vi "AuMT8852B Script Name.vi"(5 "Name (\"\")":string, 7 "Set/Get (Set)":enum16{"Set", "Get"}(ring), 8 "error in (no error)":errorcluster, 10 "Script (3)":i32=1, 11 "VISA session":refnum<visa-resource-name>) -> (0 "error out":errorcluster, 2 "error code":i32, 3 "VISA session out":refnum<visa-resource-name>, 4 "Name out":string)   [LabVIEW 2017]
doc: "Anritsu MT8852B Bluetooth Tester\n\nSets the script's display name.\n\nINPUTS\nSet/Get - whether the value is being sent to or retrieved from the instrument.\nScript - which script's name is being written or read. Scripts 1 and 2 are read-only; 3-10 are read-write.\nName - name (16 characters or less) to assign to the script.\n\nOUTPUTS\nName out - the script's current name."
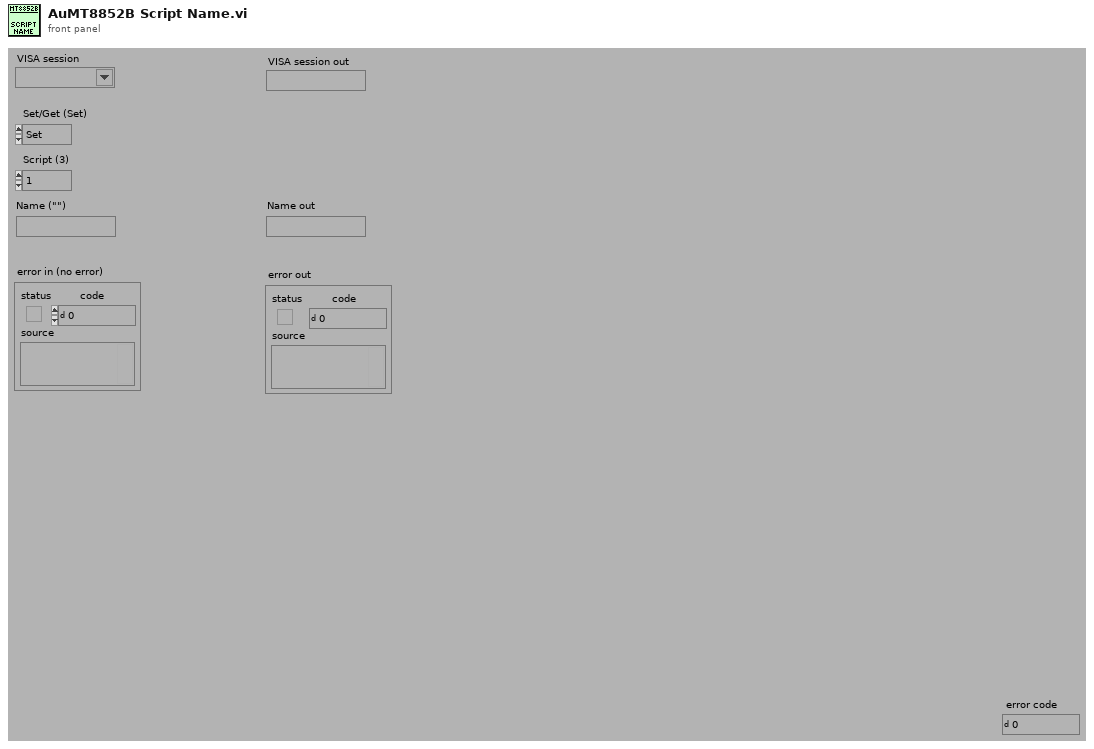
[diagram p1: front panel]
types:
  T1 = enum16{"Simulate", "Range check", "Cache", "Query instrument status"}
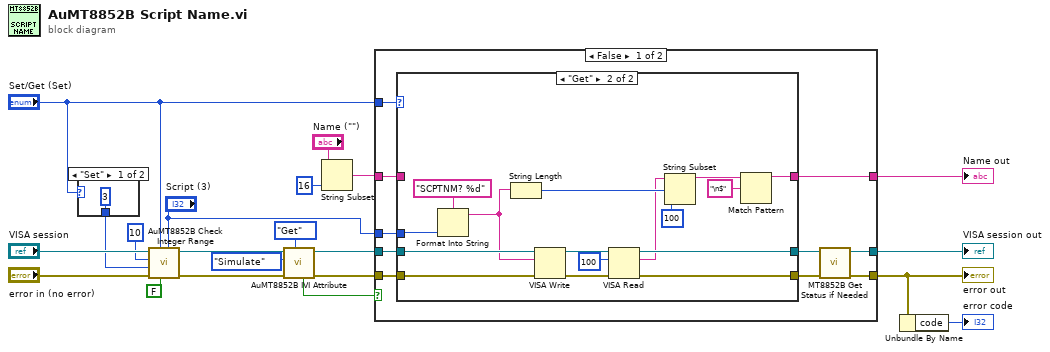
[diagram p0: block diagram]
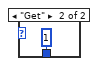
[diagram p2: hidden frame]
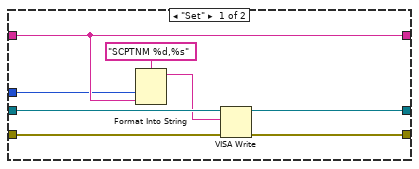
[diagram p3: hidden frame]
diagram:
  n1 = case shown="\"Set\"" "Set/Get (Set)" {
    tunnel: [3 1] -> w16
    frame "Set" {
    }
    frame "Get" {
    }
  }
  n2 = call <instrlib>:"AuMT8852B Check Integer Range.vi"("Value (0)"="Script (3)", "Check IVI flag first? (T)"=FALSE, "Set/Get (Set)"="Set/Get (Set)", "error in (no error)"="error in (no error)", "Lower limit (-1)"=w16, "Upper limit (1)"=10, "VISA session"="VISA session") -> ("error out"=w12:errorcluster, "VISA session out"=w15:refnum<visa-resource-name>)  [unwired: 3 in]
  n3 = call <instrlib>:"AuMT8852B IVI Attribute.vi"("Set/Get (Set)"=enum16{"Set", "Get"}."Get", "error in (no error)"=w12, "Flag (Simulate)"=T1."Simulate", "VISA session"=w15) -> ("error out"=w13:errorcluster, "VISA session out"=w14:refnum<visa-resource-name>, "Value out"=w9:bool)  [unwired: 5 in]
  n4 = String Subset(string="Name (\"\")", length (rest)=16 ("length (rest)")) -> (substring=w6:string)  [unwired: 1 in]
  n5 = case shown="False" w9 {
    tunnel: "Set/Get (Set)" -> [w33 _]
    tunnel: w6 -> [w32 w60]
    tunnel: [w25 w58] -> w2
    tunnel: [w26 w59] -> w21
    tunnel: w14 -> [w31 w59]
    tunnel: w13 -> [w30 w58]
    tunnel: [w29 w60] -> w20
    tunnel: "Script (3)" -> [w24 _]
    frame False {
      n6 = case shown="\"Get\"" w33 {
        tunnel: [w38 w51] -> w27
        tunnel: w32 -> [w35 _]
        tunnel: [w39 w52] -> w28
        tunnel: w31 -> [w41 w57]
        tunnel: w30 -> [w40 w56]
        tunnel: [w35 w43] -> w29
        tunnel: w24 -> [w34 w49]
        frame "Set" {
          n7 = Format Into String(format string="SCPTNM %d,%s" ("Format String"), w34, w35) -> (resulting string=w36:string)  [unwired: 2 in, 1 out]
          n8 = VISA Write(VISA resource name=w41, write buffer=w36, error in (no error)=w40) -> (VISA resource name out=w39:refnum<visa-resource-name>, error out=w38:errorcluster)  [unwired: 1 out]
        }
        frame "Get" {
          n9 = Format Into String(format string="SCPTNM? %d" ("Format String"), w49) -> (resulting string=w47:string)  [unwired: 2 in, 1 out]
          n10 = String Length(string=w47) -> (length=w46:i32)
          n11 = VISA Write(VISA resource name=w57, write buffer=w47, error in (no error)=w56) -> (VISA resource name out=w55:refnum<visa-resource-name>, error out=w53:errorcluster)  [unwired: 1 out]
          n12 = VISA Read(VISA resource name=w55, byte count=u32 100 ("byte count (0)"), error in (no error)=w53) -> (VISA resource name out=w52:refnum<visa-resource-name>, read buffer=w44:string, error out=w51:errorcluster)  [unwired: 1 out]
          n13 = String Subset(string=w44, offset (0)=w46, length (rest)=100 ("length (rest)")) -> (substring=w45:string)
          n14 = Match Pattern(string=w45, regular expression="\n$") -> (before substring=w43:string)  [unwired: 1 in, 3 out]
        }
      }
      n15 = call <instrlib>:"MT8852B Get Status if Needed.vi"("error in (no error)"=w27, "VISA session"=w28) -> ("error out"=w25:errorcluster, "VISA session out"=w26:refnum<visa-resource-name>)  [unwired: 8 in]
    }
    frame True {
    }
  }
  "error out" <- w2
  "VISA session out" <- w21
  "Name out" <- w20
  n16 = Unbundle By Name(w2) -> ("code"=→"error code":i32)
